vi "PH_Beckhoff_PP_Control.destructor.vi"(0 "i ref in":refnum<vi>, 5 "error in(no error)":errorcluster) -> (19 "error out":errorcluster)   [LabVIEW 2014, in "PH_Beckhoff_PP_Control.lvlib"]
doc: "This is the destructor of a class.\n\nLicense Agreement for this software:\n\nCopyright (C)\nGesellschaft für Schwerionenforschung, GSI\nPlanckstr. 1\n64291 Darmstadt\nGermany\n\nContact: D.Beck@gsi.de \n\nThis program is free software; you can redistribute it and/or modify it under the terms of the \nGNU General Public License as published by the Free Software Foundation; either version 2 of \nthe license, or (at your option) any later version.\n\nThis program is distributed in the hope that it will be useful, but WITHOUT ANY WARRANTY; \nwithout even the implied warranty of MERCHANTABILITY or FITNESS FOR A PARTICULAR PURPOSE. See the GNU General License for more details (http://www.gnu.org).\n\nGesellschaft für Schwerionenforschung, GSI\nPlanckstr. 1, 64291 Darmstadt, Germany\nFor all questions and ideas contact: M.Richter@gsi.de, H.Brand@gsi.de or D.Beck@gsi.de.\nLast update: 16-JUN-2004"
uses:
  PH_Beckhoff_PP_Control.lvlib
  PH_Beckhoff/PH_Beckhoff.lvlib
  CSlibraries-extern/DimLVEvent/LVDimInterface/LVDimInterface.lvlib
  CS_Core/CSSystem/CSSystemLib/CSSystemLib.lvlib
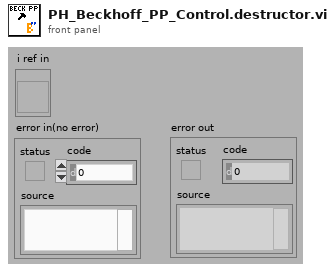
[diagram p1: front panel]
types:
  T1 = typedef "PH_Beckhoff_PP_Control.lvlib/PH_Beckhoff_PP_Control.i attribute.ctl" = cluster{"PP Conductivity Control":cluster{"PSDB":cluster{"Status Service ID":i32, "Instance ID":i32, "Data Status":T2, "Ref Status":refnum<vi>, "Error Code":i32}, "Status":cluster{"GUI Ref":refnum<vi>, "Status Service ID":i32, "Status":T3}, "DIs":cluster{"Device on":cluster{"GUI Ref":refnum<vi>, "# in Data":i32}, "Conductivity ok":cluster{"GUI Ref":refnum<vi>, "# in Data":i32}, "Temperature ok":cluster{"GUI Ref":refnum<vi>, "# in Data":i32}, "Alarm":cluster{"GUI Ref":refnum<vi>, "# in Data":i32}}, "PSDB Thread":cluster{"Ref":refnum<vi>, "Q-Ref":refnum<queue>}}, "PP Mercury Control":cluster{"PSDB":cluster{"Status Service ID":i32, "Instance ID":i32, "Data Status":T2, "Ref Status":refnum<vi>, "Error Code":i32}, "Status":cluster{"GUI Ref":refnum<vi>, "Status Service ID":i32, "Status":T3}, "on since:":cluster{"GUI Ref":refnum<vi>, "Service ID":i32, "Time":string}, "DIs":cluster{"Device on":cluster{"GUI Ref":refnum<vi>, "# in Data":i32}, "Alarm":cluster{"GUI Ref":refnum<vi>, "# in Data":i32}}, "AIs":cluster{"Concentration":cluster{"GUI Ref":refnum<vi>, "# in Data":i32}}, "PSDB Thread":cluster{"Ref":refnum<vi>, "Q-Ref":refnum<queue>}}, "PSDB":cluster{"Shot #":i32, "Subsystem":T4}, "PSDB Credentials":T5}
  T2 = typedef "PH_PSDBWriter.lvlib/PH_PSDBWriter.Data Status.ctl" = i16
  T3 = typedef "PH_StatusHandler.lvlib/PH_StatusHandler.Status.ctl" = i16
  T4 = typedef "PH_PSDBWriter.lvlib/PH_PSDBWriter.PHELIX-Subsystems.ctl" = i32
  T5 = typedef "PH_Common.lvlib/PH_Connection.PSDB Credentials.ctl" = cluster{"PW":string, "ID":string, "DS":string}
  T6 = enum16{"SetAttribute", "GetAttribute", "CreateAttribute", "DestroyAttribute", "DestroyAllAtributes"}
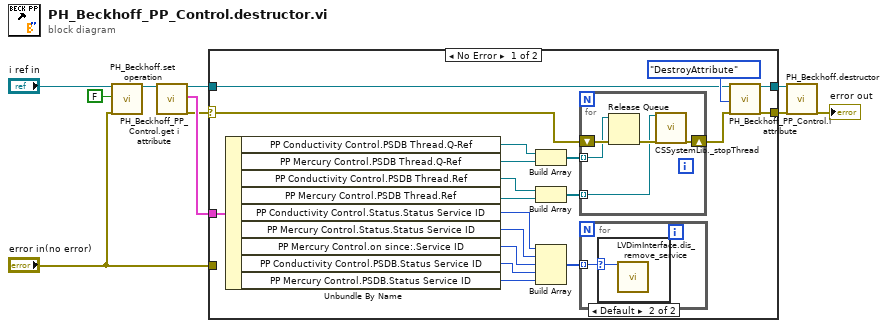
[diagram p0: block diagram]
diagram:
  n1 = call "PH_Beckhoff.set operation.vi"("VI in"="i ref in", "operation?"=FALSE, "error in (no error)"="error in(no error)") -> ("VI out"=w3:refnum<vi>)  [unwired: 15 in, 1 out]
  n2 = call "PH_Beckhoff_PP_Control.get i attribute.vi"("i ref in"=w3) -> ("i ref out"=w10:refnum<vi>, "i attribute"=w8:T1, "error out"=w7:errorcluster)  [unwired: 16 in]
  n3 = case shown="No Error" w7 {
    selector: w7 -> [w11 _]
    tunnel: w10 -> [w12 w38]
    tunnel: [w29 w38] -> w6
    tunnel: [w28 w37] -> w9
    tunnel: w8 -> [w26 _]
    tunnel: "error in(no error)" -> [_ w37]
    frame No Error {
      n4 = Unbundle By Name(w26) -> ("PP Conductivity Control.PSDB Thread.Q-Ref"=w14:refnum<queue>, "PP Mercury Control.PSDB Thread.Q-Ref"=w15:refnum<queue>, "PP Conductivity Control.PSDB Thread.Ref"=w17:refnum<vi>, "PP Mercury Control.PSDB Thread.Ref"=w18:refnum<vi>, "PP Conductivity Control.Status.Status Service ID"=w27:i32, "PP Mercury Control.Status.Status Service ID"=w24:i32, "PP Mercury Control.on since:.Service ID"=w23:i32, "PP Conductivity Control.PSDB.Status Service ID"=w22:i32, "PP Mercury Control.PSDB.Status Service ID"=w21:i32)
      n5 = Build Array(w14, w15) -> (w13:refnum<queue>[])
      n6 = Build Array(w17, w18) -> (w16:refnum<vi>[])
      n7 = Build Array(w27, w24, w23, w22, w21) -> (w25:i32[])
      n8 = for {
        shift-right: [w32] -> w19
        shift-left: w11 -> [w33]
        tunnel: w16 -> [w31] mode=indexing
        tunnel: w13 -> [w30] mode=indexing
        n9 = Release Queue(queue=w30, error in (no error)=w33) -> (error out=w34:errorcluster)  [unwired: 1 in, 2 out]
        n10 = call "CSSystemLib._stopThread.vi"("i ref in"=w31, "error in (no error)"=w34) -> ("error out"=w32:errorcluster)  [unwired: 16 in, 1 out]
      }
      n11 = for {
        tunnel: w25 -> [w35] mode=indexing
        n12 = case shown="Default" w35 {
          selector: w35 -> [_ w36]
          frame -1 {
          }
          frame Default {
            n13 = call "LVDimInterface.dis_remove_service.vi"("my_serviceID"=w36) -> ()  [unwired: 18 in, 1 out]
          }
        }
      }
      n14 = call "PH_Beckhoff_PP_Control.i attribute.vi"("VI Refnum"=w12, "Action"=T6."DestroyAttribute", "error in (no error)"=w19) -> ("VI Refnum out"=w29:refnum<vi>, "error out"=w28:errorcluster)  [unwired: 14 in, 1 out]
    }
    frame Error {
    }
  }
  n15 = call "PH_Beckhoff.destructor.vi"("i ref in"=w6, "error in(no error)"=w9) -> ("error out"=→"error out":errorcluster)  [unwired: 17 in]
